vi "Filter Names.vi"(10 "Result Filter":string, 11 "WorksheetsNames":string[](array[string])) -> (3 "Filtered":string[](array[string]))   [LabVIEW 2011]
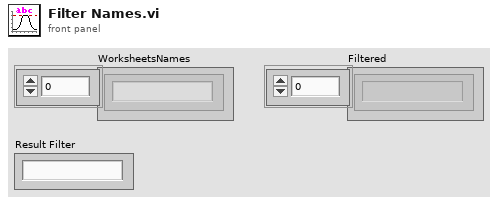
[diagram p1: front panel]
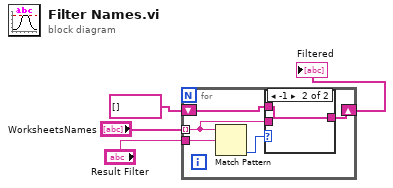
[diagram p0: block diagram]
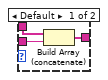
[diagram p2: hidden frame]
diagram:
  n1 = for {
    tunnel: "WorksheetsNames" -> [w6] mode=indexing
    tunnel: "Result Filter" -> [w9]
    shift-right: [w5] -> w4
    shift-left: string[] [] -> [w7]
    n2 = Match Pattern(string=w6, regular expression=w9) -> (offset past match=w8:i32)  [unwired: 1 in, 3 out]
    n3 = case shown="-1" w8 {
      tunnel: w7 -> [w12 w13]
      tunnel: w6 -> [w11 _]
      tunnel: [w10 w13] -> w5
      frame Default {
        n4 = Build Array (concatenate)(w12, w11) -> (w10:string[])
      }
      frame -1 {
      }
    }
  }
  "Filtered" <- w4
